vi "Init2000.vi"   [LabVIEW 2013]
uses:
  <vilib>/Heliosphere Research LLC/Advanced Plotting Toolkit/Advanced Plotting Toolkit.lvlib
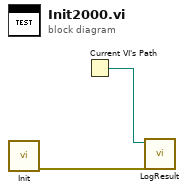
[diagram p0: block diagram]
diagram:
  n1 = call <vilib>:"Init.vi"() -> ("error out"=w1:errorcluster)  [unwired: 11 in]
  n2 = Current VI's Path() -> (path=w2:path)
  n3 = call "LogResult.vi"("Test Result"=w1, "VI Path"=w2) -> ()  [unwired: 10 in]
